vi "Temperature.vi"() -> (3 "read buffer":string)   [LabVIEW 2018]
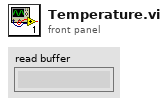
[diagram p1: front panel]
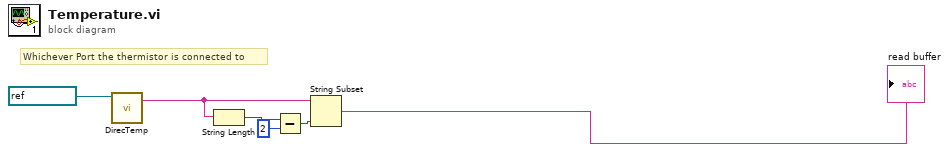
[diagram p0: block diagram]
diagram:
  # "Whichever Port the thermistor is connected to"
  n1 = call "DirecTemp.vi"("VISA resource name"=refnum<visa-resource-name> "COM10" ("DirecTemp Port")) -> ("read buffer"=w5:string)  [unwired: 3 in, 1 out]
  n2 = String Length(string=w5) -> (length=w3:i32)
  n3 = Subtract(x=w3, y=2) -> (x-y=w2:i32)
  n4 = String Subset(string=w5, length (rest)=w2) -> (substring=→"read buffer":string)  [unwired: 1 in]
